vi "XY Graph Set Plot Name Event.vi"(8 "Error In":errorcluster, 11 "Plot Name Data":T1) -> (0 "Error Out":errorcluster)   [LabVIEW 2021, in "XY Graph Add-Ons.lvlib"]
uses:
  XY Graph Add-Ons.lvlib
  XY Graph New Plot Name Data.ctl
  XY Graph Refnum.ctl
  Arrays/Arrays.lvlib
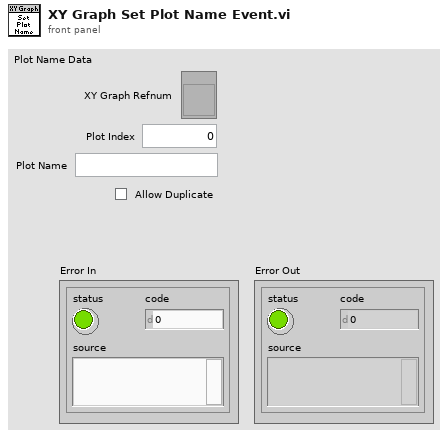
[diagram p1: front panel]
types:
  T1 = typedef "XY Graph Add-Ons.lvlib/XY Graph New Plot Name Data.ctl" = cluster{"XY Graph Refnum":T2, "Plot Index":i32, "Plot Name":string, "Allow Duplicate":bool}
  T2 = typedef "XY Graph Add-Ons.lvlib/XY Graph Refnum.ctl" = refnum<vi>
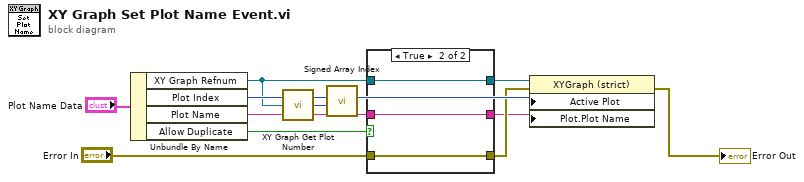
[diagram p0: block diagram]
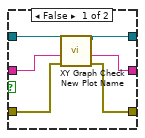
[diagram p2: hidden frame]
diagram:
  n1 = Unbundle By Name("Plot Name Data") -> ("XY Graph Refnum"=w4:T2, "Plot Index"=w11:i32, "Plot Name"=w8:string, "Allow Duplicate"=w7:bool)
  n2 = call "XY Graph Get Plot Number.vi"("XYGraph"=w4) -> ("# Plots"=w10:i32)  [unwired: 8 in]
  n3 = call "Signed Array Index.vi"("Array Size"=w10, "Array Index in"=w11) -> ("Array Index out"=w6:i32)  [unwired: 9 in]
  n4 = case shown="True" w7 {
    tunnel: w4 -> [w18 w21]
    tunnel: w8 -> [w17 w20]
    tunnel: "Error In" -> [w16 w19]
    tunnel: [w15 w21] -> w3
    tunnel: [w13 w20] -> w1
    tunnel: [w14 w19] -> w2
    frame False {
      n5 = call "XY Graph Check New Plot Name.vi"("Error In"=w16, "New Plot Name (in)"=w17, "Multiplot XY Graph Refnum in"=w18) -> ("Error Out"=w14:errorcluster, "New Plot Name (out)"=w13:string, "Multiplot XY Graph Refnum out"=w15:T2)  [unwired: 6 in]
    }
    frame True {
    }
  }
  n6 = property class="XYGraph (strict)"(reference=w3, error in=w2, "Active Plot"=w6, "Plot.Plot Name"=w1) -> (error out=→"Error Out":errorcluster)  [unwired: 1 out]
